vi "getAvailableOperationModes.vi"(8 "error in (no error)":errorcluster, 11 "IDevice in":refnum<class "IDevice.lvclass">) -> (0 "error out":errorcluster, 2 "Operation Modes out":T1[](array[typedef]) items=["daqOperationModeTypeUnknown", "daqOperationModeTypeIdle", "daqOperationModeTypeOperation", "daqOperationModeTypeSafeOperation"], 3 "IDevice out":refnum<class "IDevice.lvclass">)   [LabVIEW 2022 SP3, in "openDAQ.lvlib" / "IBaseObject.lvlib" / "IPropertyObject.lvlib" / "IComponent.lvlib" / "IFolder.lvlib" / "IDevice.lvlib" / "IDevice.lvclass"]
uses:
  <instrlib>/openDAQ/Public/Classes/IDevice/IDevice.lvclass
  <instrlib>/openDAQ/Public/Classes/IDevice/IDevice.lvclass/IDevice.ctl
  <instrlib>/openDAQ/Public/Classes/daqCoreTypes/IList/IList.lvclass
  <instrlib>/openDAQ/Binaries/Windows/x86/copendaq32.dll
  <instrlib>/openDAQ/Public/Classes/daqCoreTypes/IList/Polymorphic/getList/getIntegerList.vi
  <instrlib>/openDAQ/Public/TypeDef/daqOperationModeType.ctl
  <instrlib>/openDAQ/openDAQ.lvlib
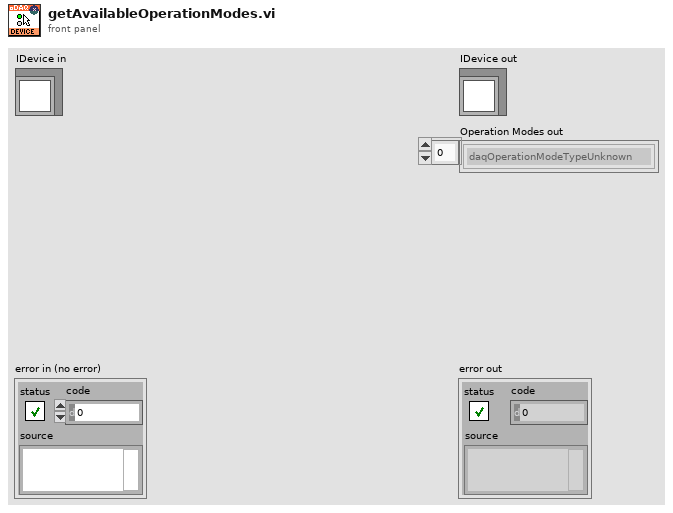
[diagram p1: front panel]
types:
  T1 = typedef "openDAQ.lvlib/daqOperationModeType.ctl" = u16
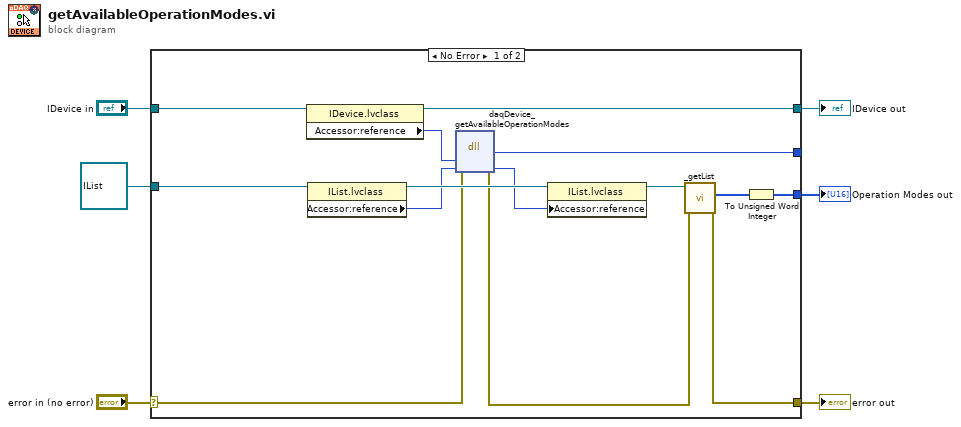
[diagram p0: block diagram]
diagram:
  n1 = case shown="No Error" "error in (no error)" {
    selector: "error in (no error)" -> [w13 w22]
    tunnel: [w8 w22] -> w5
    tunnel: [w18 w21] -> w3
    tunnel: "IDevice in" -> [w19 w21]
    tunnel: refnum<class "IList.lvclass"> refnum ("openDAQ.lvlib:daqCoreTypes.lvlib:IList.lvclass") -> [w16 _]
    tunnel: [w10 _] -> _
    tunnel: [w7 _] -> w1
    frame No Error {
      n2 = property class="IDevice.lvclass"(reference=w19) -> (reference out=w18:refnum<class "IDevice.lvclass">, "Accessor:reference"=w17:i64)  [unwired: 1 in, 1 out]
      n3 = property class="IList.lvclass"(reference=w16) -> (reference out=w20:refnum<class "IList.lvclass">, "Accessor:reference"=w15:i64)  [unwired: 1 in, 1 out]
      n4 = dll-call lib="C:/Program Files (x86)/National Instruments/LabVIEW 2022/instr.lib/openDAQ/Binaries/Windows/x86/copendaq*.*" fn="daqDevice_getAvailableOperationModes"(error in=w13, "device"=w17, "operationModes"=w15) -> (error out=w11:errorcluster, "return type"=w10:u32, "operationModes"=w14:i64)  [unwired: 3 in, 1 out]
      n5 = property class="IList.lvclass"(reference=w20, "Accessor:reference"=w14) -> (reference out=w12:refnum<class "IList.lvclass">)  [unwired: 1 in, 1 out]
      n6 = call-poly <instrlib>:"_getList.vi"("error in (no error)"=w11, "IList in"=w12) -> ("error out"=w8:errorcluster, "Integers out"=w9:i32[])  [unwired: 8 in]
      n7 = To Unsigned Word Integer(number=w9) -> (unsigned 16bit integer=w7:u16[])
    }
    frame Error {
    }
  }
  "error out" <- w5
  "IDevice out" <- w3
  "Operation Modes out" <- w1
